vi "CRYGet Cursor Info.vi"(10 "pGraph VI":refnum<vi>) -> (3 "Flattened Cursor Property":string)   [LabVIEW 2013]
uses:
  Control/CRYCursor Property.ctl
panel:
  in  "Cursor Property":T1[](array[typedef])
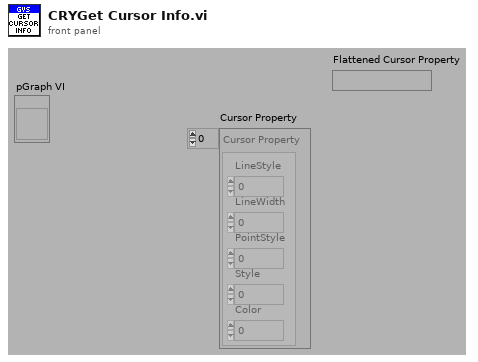
[diagram p1: front panel]
types:
  T1 = typedef "CRYCursor Property.ctl" = cluster{"LineStyle":u8, "LineWidth":u8, "PointStyle":u8, "Style":u8, "Color":u32}
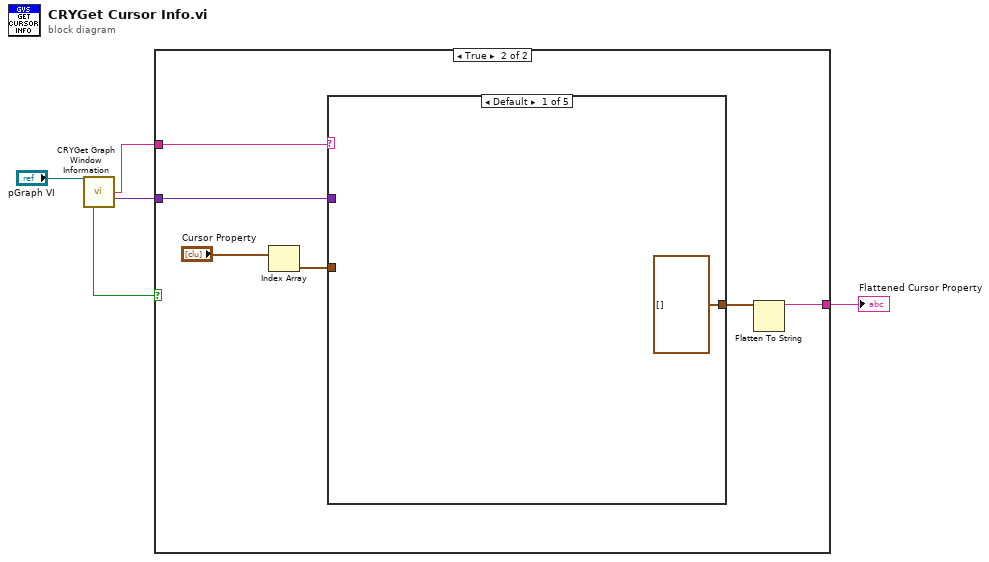
[diagram p0: block diagram]
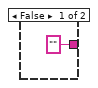
[diagram p2: hidden frame]
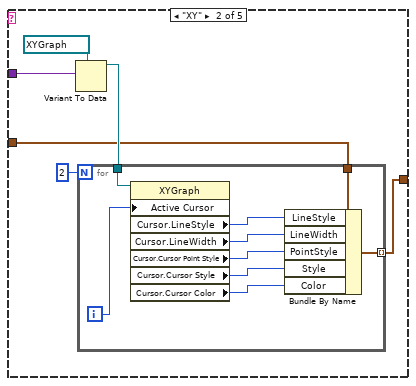
[diagram p3: hidden frame]
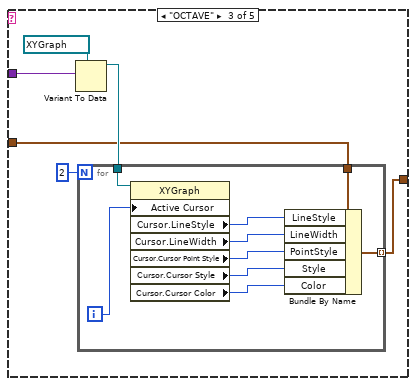
[diagram p4: hidden frame]
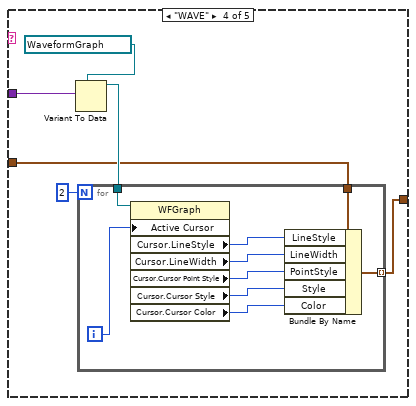
[diagram p5: hidden frame]
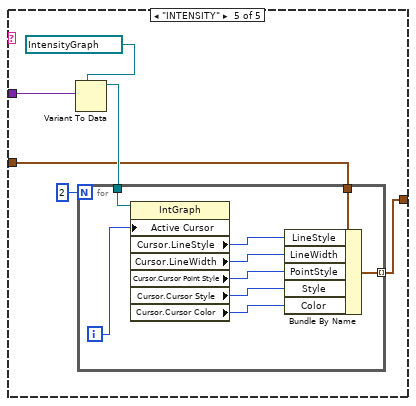
[diagram p6: hidden frame]
diagram:
  n1 = call "CRYGet Graph Window Information.vi"("pGraph VI In"="pGraph VI") -> ("Graph Type Out"=w1:string, "Graph Control Ref Out"=w2:variant, "CursorShow Out"=w4:bool)  [unwired: 4 in, 8 out]
  n2 = case shown="True" w4 {
    tunnel: w1 -> [_ w12]
    tunnel: ["" ("data string") w8] -> w5
    tunnel: w2 -> [_ w7]
    frame False {
    }
    frame True {
      n3 = Index Array(array="Cursor Property") -> (element=w10:T1)  [unwired: 1 in]
      n4 = case shown="Default" w12 {
        tunnel: w7 -> [_ w19 w34 w49 w64]
        tunnel: [T1[] [] w16 w31 w47 w62] -> w9
        tunnel: w10 -> [_ w15 w30 w46 w61]
        frame Default {
        }
        frame "XY" {
          n5 = Variant To Data(type=refnum<vi> refnum ("XY Graph"), Variant=w19) -> (data=w17:refnum<vi>)  [unwired: 1 in, 1 out]
          n6 = for {
            N: 2 -> [_]
            tunnel: w17 -> [w28]
            tunnel: w15 -> [w26]
            tunnel: [w20] -> w16 mode=indexing
            i -> [w27]
            n7 = property class="XYGraph"(reference=w28, "Active Cursor"=w27) -> ("Cursor.LineStyle"=w25:u8, "Cursor.LineWidth"=w24:u8, "Cursor.Cursor Point Style"=w23:u8, "Cursor.Cursor Style"=w22:u8, "Cursor.Cursor Color"=w21:u32)  [unwired: 1 in, 2 out]
            n8 = Bundle By Name(cluster=w26, "LineStyle"=w25, "LineWidth"=w24, "PointStyle"=w23, "Style"=w22, "Color"=w21) -> (w20:T1)
          }
        }
        frame "OCTAVE" {
          n9 = Variant To Data(type=refnum<vi> refnum ("XY Graph"), Variant=w34) -> (data=w32:refnum<vi>)  [unwired: 1 in, 1 out]
          n10 = for {
            N: 2 -> [_]
            tunnel: w32 -> [w43]
            tunnel: w30 -> [w41]
            tunnel: [w35] -> w31 mode=indexing
            i -> [w42]
            n11 = property class="XYGraph"(reference=w43, "Active Cursor"=w42) -> ("Cursor.LineStyle"=w40:u8, "Cursor.LineWidth"=w39:u8, "Cursor.Cursor Point Style"=w38:u8, "Cursor.Cursor Style"=w37:u8, "Cursor.Cursor Color"=w36:u32)  [unwired: 1 in, 2 out]
            n12 = Bundle By Name(cluster=w41, "LineStyle"=w40, "LineWidth"=w39, "PointStyle"=w38, "Style"=w37, "Color"=w36) -> (w35:T1)
          }
        }
        frame "WAVE" {
          n13 = Variant To Data(type=refnum<vi> refnum ("WaveGraph Ref"), Variant=w49) -> (data=w48:refnum<vi>)  [unwired: 1 in, 1 out]
          n14 = for {
            N: 2 -> [_]
            tunnel: w48 -> [w58]
            tunnel: w46 -> [w56]
            tunnel: [w50] -> w47 mode=indexing
            i -> [w57]
            n15 = property class="WFGraph"(reference=w58, "Active Cursor"=w57) -> ("Cursor.LineStyle"=w55:u8, "Cursor.LineWidth"=w54:u8, "Cursor.Cursor Point Style"=w53:u8, "Cursor.Cursor Style"=w52:u8, "Cursor.Cursor Color"=w51:u32)  [unwired: 1 in, 2 out]
            n16 = Bundle By Name(cluster=w56, "LineStyle"=w55, "LineWidth"=w54, "PointStyle"=w53, "Style"=w52, "Color"=w51) -> (w50:T1)
          }
        }
        frame "INTENSITY" {
          n17 = Variant To Data(type=refnum<vi> refnum ("WaveGraph Ref"), Variant=w64) -> (data=w63:refnum<vi>)  [unwired: 1 in, 1 out]
          n18 = for {
            N: 2 -> [_]
            tunnel: w63 -> [w73]
            tunnel: w61 -> [w71]
            tunnel: [w65] -> w62 mode=indexing
            i -> [w72]
            n19 = property class="IntGraph"(reference=w73, "Active Cursor"=w72) -> ("Cursor.LineStyle"=w70:u8, "Cursor.LineWidth"=w69:u8, "Cursor.Cursor Point Style"=w68:u8, "Cursor.Cursor Style"=w67:u8, "Cursor.Cursor Color"=w66:u32)  [unwired: 1 in, 2 out]
            n20 = Bundle By Name(cluster=w71, "LineStyle"=w70, "LineWidth"=w69, "PointStyle"=w68, "Style"=w67, "Color"=w66) -> (w65:T1)
          }
        }
      }
      n21 = Flatten To String(anything=w9) -> (data string=w8:string)  [unwired: 3 in, 2 out]
    }
  }
  "Flattened Cursor Property" <- w5
